vi "Inititalize.vi"(7 "Active measurement":string, 8 "error in":errorcluster, 10 "Trigger edge":T1=1800 items=["Rising Edge"=1800, "Falling Edge"=1801], 11 "DPI resource name":string) -> (0 "error out":errorcluster, 2 "DPI Bitfile reference":refnum<k20>, 3 "DPI Session":refnum<k15>)   [LabVIEW 2021, in "dcvmDPI_AD7606B_serverImpl.lvlib"]
uses:
  dcvmDPI_AD7606B_serverImpl.lvlib
  <instrlib>/niDigital/niDigital.llb/niDigital Trigger Digital Edge - Edge.ctl
  <instrlib>/niDigital/niDigital.llb/niDigital Export Signal.ctl
  <instrlib>/niDigital/niDigital.llb/niDigital Conditional Jump Trigger ID.ctl
  <vilib>/Utility/error.llb/Error Cluster From Error Code.vi
  <vilib>/rvi/errors/niLvFpgaAdjustHostInterfaceError.vi
  <instrlib>/niDigital/niDigital.llb/niDigital Load Specifications Levels and Timing (Multiple).vi
  <instrlib>/niDigital/niDigital.llb/niDigital Configure Digital Edge Conditional Jump Trigger.vi
  <instrlib>/niDigital/niDigital.llb/niDigital Create Capture Waveform (Parallel).vi
  <vilib>/rvi/interface/nirviReadWriteControl/nirviReadWriteControl.xnode
  NiFpgaLv.dll
  <vilib>/rvi/interface/Simulation/niFpgaSimulationCallBeginRW.vi
panel:
  in  "Pin config":T2(array[cluster])=[{"Pin"="RESET", "Current Limit"=0.01, "Voltage Level"=3.3}, {"Pin"="SCLK", "Current Limit"=0.01, "Voltage Level"=3.3}, {"Pin"="CS", "Current Limit"=0.01, "Voltage Level"=3.3}, {"Pin"="WR", "Current Limit"=0.01, "Voltage Level"=3.3}, {"Pin"="CONVST", "Current Limit"=0.01, "Voltage Level"=0.0}, {"Pin"="REFSEL", "Current Limit"=0.01, "Voltage Level"=3.3}, {"Pin"="STBY", "Current Limit"=0.01, "Voltage Level"=3.3}, {"Pin"="SERPAR", "Current Limit"=0.01, "Voltage Level"=0.0}, {"Pin"="RANGE", "Current Limit"=0.01, "Voltage Level"=0.0}, {"Pin"="OS0", "Current Limit"=0.01, "Voltage Level"=0.0}, {"Pin"="OS1", "Current Limit"=0.01, "Voltage Level"=0.0}, {"Pin"="OS2", "Current Limit"=0.01, "Voltage Level"=0.0}, {"Pin"="RESET", "Current Limit"=0.01, "Voltage Level"=0.0}]
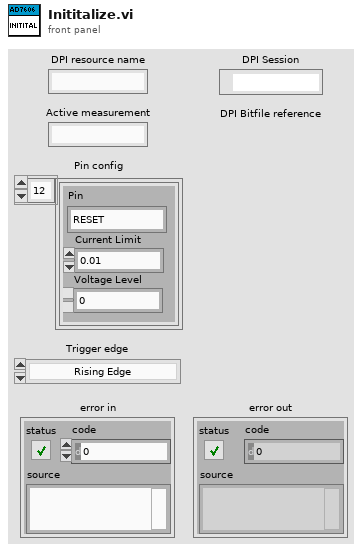
[diagram p1: front panel]
types:
  T1 = typedef "niDigital Trigger Digital Edge - Edge.ctl" = i32
  T2 = cluster{"Pin":string, "Current Limit":dbl, "Voltage Level":dbl}[]
  T3 = typedef "niDigital Conditional Jump Trigger ID.ctl" = string
  T4 = cluster{"high pins":string, "low pins":string, "tristate pins":string}
  T5 = typedef "niDigital Export Signal.ctl" = i32
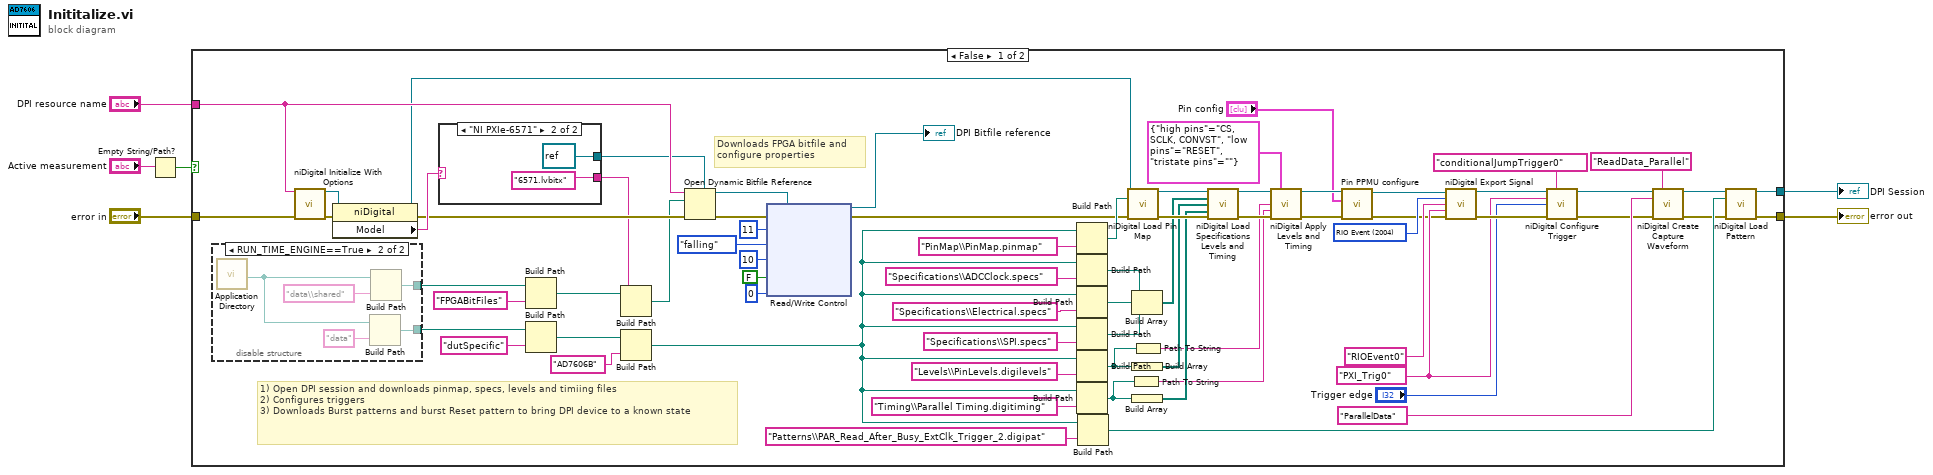
[diagram p0: block diagram]
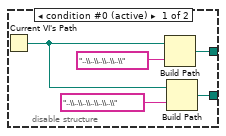
[diagram p2: hidden frame]
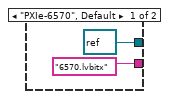
[diagram p3: hidden frame]
diagram:
  n1 = Empty String/Path?(string/path="Active measurement") -> (empty?=w1:bool)
  n2 = case shown="False" w1 {
    tunnel: "DPI resource name" -> [w77 _]
    tunnel: "error in" -> [w75 w92]
    tunnel: [w16 w92] -> w4
    tunnel: [w15 _] -> w3
    frame False {
      w34 = "PXI_Trig0" ("output terminal")
      w37 = T5 2004 items=["Start Trigger"=2000, "Conditional Jump Trigger"=2001, "Pattern Opcode Event"=2002, "RIO Event"=2004] ("signal")
      # "1) Open DPI session and downloads pinmap, specs, levels and timiing files\n2) Configures triggers\n3) Downloads Burst patterns and burst Reset pattern to bring DPI device to a known state"
      # "Downloads FPGA bitfile and\nconfigure properties"
      n3 = disable-structure shown="RUN_TIME_ENGINE==True" {
        disable-tunnel: [w82 w86] -> w8
        disable-tunnel: [w80 w85] -> w7
        frame condition #0 (active) {
          n4 = Current VI's Path() -> (path=w81:path)
          n5 = Build Path(base path=w81, name or relative path="..\\..\\..\\..\\..\\") -> (appended path=w82:path)
          n6 = Build Path(base path=w81, name or relative path="..\\..\\..\\..\\..\\..\\") -> (appended path=w80:path)
        }
        frame condition #1 {
          n7 = call <vilib>:"Application Directory.vi"() -> ("Application Directory"=w84:path)
          n8 = Build Path(base path=w84, name or relative path="data") -> (appended path=w85:path)
          n9 = Build Path(base path=w84, name or relative path="data\\shared") -> (appended path=w86:path)
        }
      }
      n10 = call <instrlib>:"niDigital Initialize With Options.vi"("resource name"=w77, "error in"=w75) -> ("instrument handle"=w73:refnum<k15>, "error out"=w72:errorcluster)  [unwired: 12 in]
      n11 = property on="Property Node" class="niDigital"(reference=w73, error in=w72) -> (reference out=w18:refnum<k15>, error out=w74:errorcluster, "Model"=w76:string)
      n12 = case shown="\"NI PXIe-6571\"" w76 {
        tunnel: [refnum<k20> refnum ("Type") refnum<k20> refnum ("Type")] -> w61
        tunnel: ["6570.lvbitx" ("element") "6571.lvbitx" ("element")] -> w71
        frame "PXIe-6570", Default {
        }
        frame "NI PXIe-6571" {
        }
      }
      n13 = Build Path(base path=w8, name or relative path="FPGABitFiles") -> (appended path=w13:path)
      n14 = Build Path(base path=w7, name or relative path="dutSpecific") -> (appended path=w11:path)
      n15 = Build Path(base path=w13, name or relative path=w71) -> (appended path=w70:path)
      n16 = Build Path(base path=w11, name or relative path="AD7606B" ("dutName")) -> (appended path=w9:path)
      n17 = Open Dynamic Bitfile Reference(0:w77, 1:w70, 3:w74, 4:w61) -> (5:w63:refnum<k20>, 8:w62:errorcluster)  [unwired: 1 in]
      n18 = xnode "Read/Write Control"("FPGA VI Reference In"=w63, "error in"=w62, "trigger line"=11, "edge"=enum16{"rising", "falling"}."falling", "holdoff time"=u16 10, "active"=FALSE, "delay"=u8 0) -> ("FPGA VI Reference Out"=→"DPI Bitfile reference":refnum<k20>, "error out"=w19:errorcluster)
      n19 = Build Path(base path=w9, name or relative path="PinMap\\PinMap.pinmap" ("element")) -> (appended path=w59:path)
      n20 = Build Path(base path=w9, name or relative path="Specifications\\ADCClock.specs" ("element")) -> (appended path=w50:path)
      n21 = Build Path(base path=w9, name or relative path="Specifications\\Electrical.specs" ("element")) -> (appended path=w51:path)
      n22 = Build Path(base path=w9, name or relative path="Specifications\\SPI.specs" ("element")) -> (appended path=w52:path)
      n23 = Build Path(base path=w9, name or relative path="Levels\\PinLevels.digilevels" ("element")) -> (appended path=w44:path)
      n24 = Build Path(base path=w9, name or relative path="Timing\\Parallel Timing.digitiming" ("element")) -> (appended path=w43:path)
      n25 = Build Path(base path=w9, name or relative path="Patterns\\PAR_Read_After_Busy_ExtClk_Trigger_2.digipat" ("element")) -> (appended path=w28:path)
      n26 = call <instrlib>:"niDigital Load Pin Map.vi"("instrument handle"=w18, "pin map file"=w59, "error in"=w19) -> ("instrument handle out"=w58:refnum<k15>, "error out"=w57:errorcluster)  [unwired: 11 in]
      n27 = Path To String(path=w43) -> (string=w42:string)
      n28 = Build Array(w50, w51, w52) -> (w49:path[])
      n29 = Build Array(w44) -> (w48:path[])
      n30 = Build Array(w43) -> (w47:path[])
      n31 = Path To String(path=w44) -> (string=w41:string)
      n32 = call-poly <instrlib>:"niDigital Load Specifications Levels and Timing.vi"("instrument handle"=w58, "specifications file paths"=w49, "levels file paths"=w48, "timing file paths"=w47, "error in"=w57) -> ("instrument handle out"=w46:refnum<k15>, "error out"=w45:errorcluster)  [unwired: 9 in]
      n33 = call <instrlib>:"niDigital Apply Levels and Timing.vi"("instrument handle"=w46, "initial state"=T4 {"high pins"="CS, SCLK, CONVST", "low pins"="RESET", "tristate pins"=""}, "levels sheet"=w41, "timing sheet"=w42, "error in"=w45) -> ("instrument handle out"=w23:refnum<k15>, "error out"=w21:errorcluster)  [unwired: 9 in]
      n34 = call "Pin PPMU configure.vi"("error in (no error)"=w21, "Pin config"="Pin config", "IVI Refnum in"=w23) -> ("error out"=w20:errorcluster, "IVI Refnum out"=w22:refnum<k15>)  [unwired: 7 in]
      n35 = call <instrlib>:"niDigital Export Signal.vi"("instrument handle"=w22, "signal"=w37, "signal ID"="RIOEvent0" ("element"), "output terminal"=w34, "error in"=w20) -> ("instrument handle out"=w39:refnum<k15>, "error out"=w38:errorcluster)  [unwired: 9 in]
      n36 = call-poly <instrlib>:"niDigital Configure Trigger.vi"("instrument handle"=w39, "trigger ID"=T3 "conditionalJumpTrigger0", "source"=w34, "edge"="Trigger edge", "error in"=w38) -> ("instrument handle out"=w31:refnum<k15>, "error out"=w30:errorcluster)  [unwired: 9 in]
      n37 = call-poly <instrlib>:"niDigital Create Capture Waveform.vi"("instrument handle"=w31, "waveform name"="ReadData_Parallel" ("pin list"), "pin list"="ParallelData", "error in"=w30) -> ("instrument handle out"=w27:refnum<k15>, "error out"=w26:errorcluster)  [unwired: 10 in]
      n38 = call <instrlib>:"niDigital Load Pattern.vi"("instrument handle"=w27, "pattern file"=w28, "error in"=w26) -> ("instrument handle out"=w15:refnum<k15>, "error out"=w16:errorcluster)  [unwired: 11 in]
    }
    frame True {
    }
  }
  "DPI Session" <- w3
  "error out" <- w4
